vi "Send Connection.vi"(5 "Parameters":variant, 6 "Timeout":i32=5000, 7 "Message Priority (Normal)":T1=enum."Normal", 8 "error in (no error)":errorcluster, 9 "Port":u16=102, 10 "IP Address":string, 11 "Message Enqueuer":refnum<class "Message Enqueuer.lvclass">) -> (0 "error out":errorcluster, 3 "Message Enqueuer out":refnum<class "Message Enqueuer.lvclass">)   [LabVIEW 2025, in "PLC_Abstr.lvlib" / "Connection Msg.lvclass"]
doc: "This VI sends the message to an actor."
uses:
  Connection Msg.lvclass
  <vilib>/ActorFramework/Message Enqueuer/Message Enqueuer.lvclass
  <vilib>/ActorFramework/Message Enqueuer/Message Priority.ctl
  Connection Msg.lvclass/Connection Msg.ctl
  <vilib>/ActorFramework/Message Enqueuer/Message Enqueuer.lvclass/Message Enqueuer.ctl
  <vilib>/ActorFramework/Message Priority Queue/Priority Enqueue.vi
  C:/Program Files (x86)/National Instruments/LabVIEW 2025/vi.lib/ActorFramework/Message/Message.lvclass
  D:/Hardware/PLC/PLC_Abstr/PLC_Abstr Messages/Connection Msg/Connection Msg.lvclass
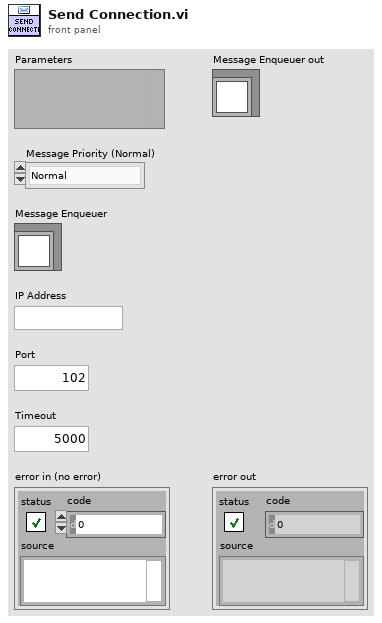
[diagram p1: front panel]
types:
  T1 = typedef "Actor Framework.lvlib/Message Enqueuer.lvclass/Message Priority.ctl" = enum16{"Low", "Normal", "High"}
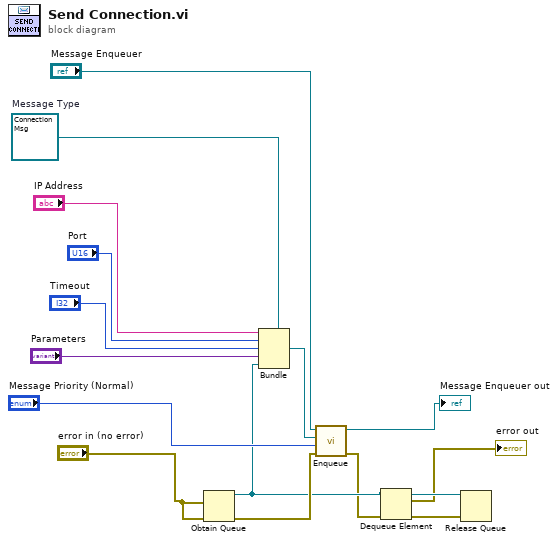
[diagram p0: block diagram]
diagram:
  w15 = refnum<class "Connection Msg.lvclass"> refnum  # Message Type
  n1 = Obtain Queue(element data type="error in (no error)", error in (no error)="error in (no error)") -> (queue out=w5:refnum<queue>, error out=w6:errorcluster)  [unwired: 3 in, 1 out]
  n2 = Bundle(cluster=w15, "IP Address", "Port", "Timeout", "Parameters", w5) -> (w14:refnum<class "Connection Msg.lvclass">)
  n3 = call <vilib>:"Enqueue.vi"("error in (no error)"=w6, "Message Priority (Normal)"="Message Priority (Normal)", "Message"=w14, "Message Enqueuer in"="Message Enqueuer") -> ("error out"=w4:errorcluster, "Message Enqueuer out"=→"Message Enqueuer out":refnum<class "Message Enqueuer.lvclass">)  [unwired: 6 in]
  n4 = Dequeue Element(queue=w5, error in (no error)=w4) -> (queue out=w3:refnum<queue>, element=→"error out":errorcluster, error out=w2:errorcluster)  [unwired: 1 in, 1 out]
  n5 = Release Queue(queue=w3, error in (no error)=w2) -> ()  [unwired: 1 in, 3 out]
